vi "esp301 set position.vi"(7 "String":string, 8 "error in (no error)":errorcluster, 9 "Args":string[](array[string]), 10 "Seperator in":string, 11 "ESP301 in":refnum<class "ESP301.lvclass">) -> (0 "error out":errorcluster, 1 "s/mm":dbl=2.0, 2 "new commands":string, 3 "ESP301 out":refnum<class "ESP301.lvclass">, 5 "timeout":dbl)   [LabVIEW 2020, in "ESP301.lvclass"]
uses:
  ESP301.lvclass
  OnOffTypeDef.ctl
  ESP301.lvclass/ESP301.ctl
  openg_time.lvlib
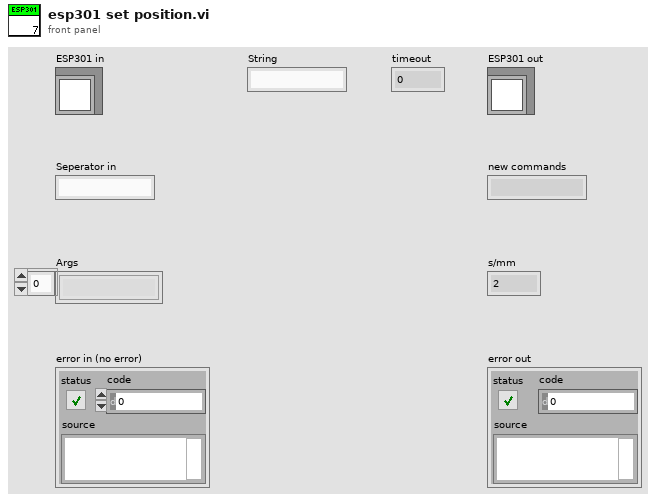
[diagram p1: front panel]
types:
  T1 = typedef "OnOffTypeDef.ctl" = enum16{"off", "on"}
  T2 = typedef "ESP301.lvclass/SettingsTypdef.ctl" = cluster{"devport":string, "Position":cluster{"Axis 1":cluster{"Value":dbl, "Min":dbl, "Max":dbl, "StepSize":dbl, "Tolerance":dbl, "ValueActual":dbl}, "Axis 2":cluster{"Value":dbl, "Min":dbl, "Max":dbl, "StepSize":dbl, "Tolerance":dbl, "ValueActual":dbl}, "Axis 3":cluster{"Value":dbl, "Min":dbl, "Max":dbl, "StepSize":dbl, "Tolerance":dbl, "ValueActual":dbl}}, "Power":cluster{"Axis 1":T1, "Axis 2":T1, "Axis 3":T1}, "Status":cluster{"Axis 1":T3, "Axis 2":T3, "Axis 3":T3}, "Backlash":cluster{"Axis 1":cluster{"Value":dbl, "Min":dbl, "Max":dbl, "StepSize":dbl, "Tolerance":dbl, "ValueActual":dbl}, "Axis 2":cluster{"Value":dbl, "Min":dbl, "Max":dbl, "StepSize":dbl, "Tolerance":dbl, "ValueActual":dbl}, "Axis 3":cluster{"Value":dbl, "Min":dbl, "Max":dbl, "StepSize":dbl, "Tolerance":dbl, "ValueActual":dbl}}, "Home":cluster{"Axis 1":cluster{"Value":dbl, "Min":dbl, "Max":dbl, "StepSize":dbl, "Tolerance":dbl, "ValueActual":dbl}, "Axis 2":cluster{"Value":dbl, "Min":dbl, "Max":dbl, "StepSize":dbl, "Tolerance":dbl, "ValueActual":dbl}, "Axis 3":cluster{"Value":dbl, "Min":dbl, "Max":dbl, "StepSize":dbl, "Tolerance":dbl, "ValueActual":dbl}}, "MoveToHardLimit":cluster{"Axis 1":T4, "Axis 2":T4, "Axis 3":T4}, "relativeMove":cluster{"Axis 1neg":T1, "Axis 2neg":T1, "Axis 3neg":T1, "Axis 1pos":T1, "Axis 2pos":T1, "Axis 3pos":T1}, "stepsize":cluster{"Value":dbl, "Min":dbl, "Max":dbl, "StepSize":dbl, "Tolerance":dbl, "ValueActual":dbl}, "automotoroff":T1, "ResetBeforeMove":T1, "Enable":cluster{"Axis 1":T1, "Axis 2":T1, "Axis 3":T1}}
  T3 = typedef "status_TypDef.ctl" = enum16{"Not referenced", "Homing", "Moving", "Ready"}
  T4 = typedef "Hardware limit.ctl" = enum16{"pos", "neg"}
  T5 = cluster{"Axis 1":cluster{"Value":dbl, "Min":dbl, "Max":dbl, "StepSize":dbl, "Tolerance":dbl, "ValueActual":dbl}, "Axis 2":cluster{"Value":dbl, "Min":dbl, "Max":dbl, "StepSize":dbl, "Tolerance":dbl, "ValueActual":dbl}, "Axis 3":cluster{"Value":dbl, "Min":dbl, "Max":dbl, "StepSize":dbl, "Tolerance":dbl, "ValueActual":dbl}}
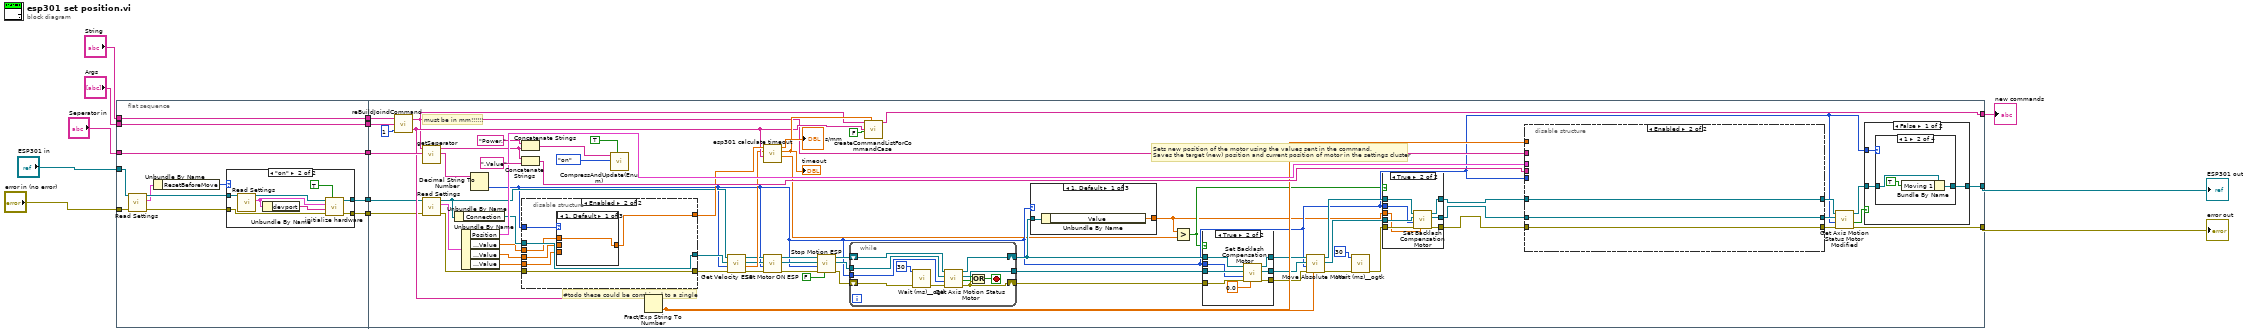
[diagram p0: block diagram]
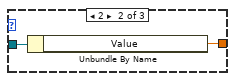
[diagram p3: hidden frame]
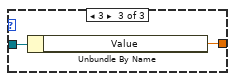
[diagram p4: hidden frame]
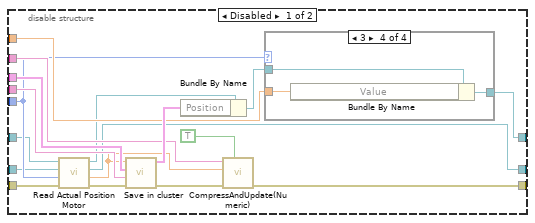
[diagram p7: hidden frame]
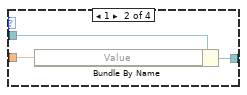
[diagram p9: hidden frame]
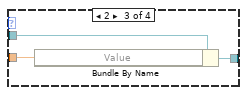
[diagram p10: hidden frame]
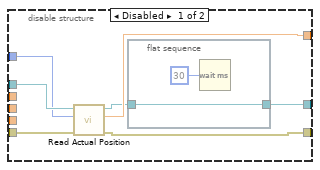
[diagram p11: hidden frame]
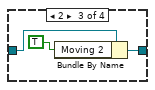
[diagram p15: hidden frame]
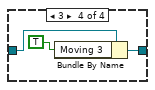
[diagram p16: hidden frame]
diagram:
  n1 = flat-sequence {
    tunnel: "error in (no error)" -> [w15]
    tunnel: "ESP301 in" -> [w14]
    tunnel: "Seperator in" -> [w22]
    tunnel: "String" -> [w23]
    tunnel: "Args" -> [w24]
    tunnel: [w24] -> w13
    tunnel: [w23] -> w12
    tunnel: [w22] -> w11
    tunnel: [w21] -> w10
    tunnel: [w20] -> w9
    tunnel: [w102] -> w1
    tunnel: [w61] -> w2
    tunnel: [w94] -> w6
    tunnel: w13 -> [w100]
    tunnel: w12 -> [w99]
    tunnel: w11 -> [w98]
    tunnel: w10 -> [w56]
    tunnel: w9 -> [w54]
    frame #0 {
      n2 = call-dynamic "Read Settings.vi"("error in (no error)"=w15, "ESP301 in"=w14) -> ("error out"=w16:errorcluster, "Settings"=w17:T2, "ESP301 out"=w18:refnum<class "ESP301.lvclass">)  [unwired: 7 in]
      n3 = Unbundle By Name(w17) -> ("ResetBeforeMove"=w19:T1)
      n4 = case shown="\"on\"" w19 {
        tunnel: [w26 w34] -> w21
        tunnel: w18 -> [w26 w29]
        tunnel: w16 -> [w25 w32]
        tunnel: [w25 w31] -> w20
        frame "off", Default {
        }
        frame "on" {
          n5 = call-dynamic "Read Settings.vi"("ESP301 in"=w29) -> ("Settings"=w27:T2, "ESP301 out"=w28:refnum<class "ESP301.lvclass">)  [unwired: 8 in, 1 out]
          n6 = Unbundle By Name(w27) -> ("devport"=w33:string)
          n7 = call-dynamic "initialize hardware.vi"("Reset (False)"=TRUE, "error in (no error)"=w32, "devport"=w33, "Settings"=w27, "ESP301 in"=w28) -> ("error out"=w31:errorcluster, "ESP301 out"=w34:refnum<class "ESP301.lvclass">)  [unwired: 4 in, 1 out]
        }
      }
    }
    frame #1 {
      # "#todo these could be combined to a single"
      # "must be in mm!!!!!!"
      # "Sets new position of the motor using the values sent in the command.\nSaves the target (new) position and current position of motor in the settings cluster"
      n8 = call "reBuildJoindCommand.vi"("number of group elements (0)"=1, "Args"=w100, "Command 2"=w99) -> ("Arg"=w82:string, "Command"=w81:string)
      n9 = call "getSeperator.vi"("Channel Seperator (\"\")"=w98, "Command"=w81) -> ("Channel"=w97:string, "Seperator (e.g. \"Channel1\")"=w89:string)  [unwired: 8 in]
      n10 = call-dynamic "Read Settings.vi"("error in (no error)"=w54, "ESP301 in"=w56) -> ("error out"=w55:errorcluster, "Settings"=w58:T2, "ESP301 out"=w57:refnum<class "ESP301.lvclass">)  [unwired: 7 in]
      n11 = Unbundle By Name(w57) -> ("Connection"=w85:refnum<visa-resource-name>)
      n12 = Unbundle By Name(w58) -> ("Position"=w92:T5, "Position.Axis 1.Value"=w53:dbl, "Position.Axis 2.Value"=w52:dbl, "Position.Axis 3.Value"=w51:dbl)
      n13 = Decimal String To Number(string=w97) -> (number=w41:i32)  [unwired: 2 in, 1 out]
      n14 = Concatenate Strings("Power." ("string"), w89) -> (w88:string)
      n15 = Concatenate Strings(w89, ".Value" ("string")) -> (w95:string)
      n16 = disable-structure shown="Enabled" {
        disable-tunnel: w85 -> [w168 w177]
        disable-tunnel: [w167 w175] -> w84
        disable-tunnel: [w162 w177] -> w79
        disable-tunnel: w55 -> [w166 w171]
        disable-tunnel: [w165 w171] -> w80
        disable-tunnel: w41 -> [w164 w176]
        disable-tunnel: w53 -> [_ w174]
        disable-tunnel: w52 -> [_ w173]
        disable-tunnel: w51 -> [_ w172]
        frame Disabled {
          n17 = call "Read Actual Position.vi"("error in (no error)"=w166, "Axis (1)"=w164, "VISA resource name"=w168) -> ("error out"=w165:errorcluster, "Position (units)"=w167:dbl, "VISA resource name out"=w163:refnum<visa-resource-name>)  [unwired: 2 in]
          n18 = flat-sequence {
            tunnel: w163 -> [w170]
            tunnel: [w170] -> w162
            frame #0 {
              n19 = Wait (ms)(milliseconds to wait=u32 30) -> ()  [unwired: 1 out]
            }
          }
        }
        frame Enabled {
          n20 = case shown="1, Default" w176 {
            tunnel: [w178 w179 w180] -> w175
            tunnel: w174 -> [w178 _ _]
            tunnel: w173 -> [_ w179 _]
            tunnel: w172 -> [_ _ w180]
            frame 1, Default {
            }
            frame 2 {
            }
            frame 3 {
            }
          }
        }
      }
      n21 = call "CompressAndUpdate(Enum).vi"("force CVT update (false)"=TRUE ("force CVT update"), "enum variant"=OnOffTypeDef."on" ("Axis 1"), "command or variable name"=w88) -> ()  [unwired: 8 in, 1 out]
      n22 = Fract/Exp String To Number(string=w82) -> (number=w67:dbl)  [unwired: 3 in, 1 out]
      n23 = call-dynamic "Get Velocity ESP.vi"("error in (no error)"=w80, "Axis (1)"=w41, "VISA resource name"=w79, "ESP301 in"=w57) -> ("error out"=w75:errorcluster, "Velocity (units/s)"=w78:dbl, "VISA resource name out"=w76:refnum<visa-resource-name>, "ESP301 out"=w77:refnum<class "ESP301.lvclass">)  [unwired: 4 in]
      n24 = call "esp301 calculate timeout.vi"("Arg"=w82, "Velocity (units/s)"=w78, "Position (units)"=w84) -> ("distance to move"=w40:dbl, "Numeric"=w83:dbl, "Numeric 2"=→"s/mm":dbl)  [unwired: 6 in]
      "timeout" <- w83
      n25 = call-dynamic "Set Motor ON ESP.vi"("error in (no error)"=w75, "Axis (1)"=w41, "VISA resource name"=w76, "ESP301 in"=w77) -> ("error out"=w74:errorcluster, "VISA resource name out"=w72:refnum<visa-resource-name>, "ESP301 out"=w69:refnum<class "ESP301.lvclass">)  [unwired: 5 in]
      n26 = call-dynamic "Stop Motion ESP.vi"("Stop all axes (F)"=FALSE, "error in (no error)"=w74, "Axis (1)"=w41, "VISA resource name"=w72, "ESP301 in"=w69) -> ("error out"=w70:errorcluster, "VISA resource name out"=w71:refnum<visa-resource-name>, "ESP301 out"=w68:refnum<class "ESP301.lvclass">)  [unwired: 4 in]
      n27 = while {
        tunnel: w71 -> [w204]
        tunnel: w41 -> [w200]
        tunnel: [w197] -> w49
        shift-right: [w202] -> w47
        shift-left: w70 -> [w203]
        shift-right: [w198] -> w42
        shift-left: w68 -> [w199]
        stop <- w205 stop-if-true
        n28 = call "Wait (ms)__ogtk.vi"("error in (no error)"=w203, "milliseconds to wait"=u32 30) -> ("error out"=w196:errorcluster)  [unwired: 8 in, 1 out]
        n29 = call-dynamic "Get Axis Motion Status Motor.vi"("error in (no error)"=w196, "Axis (1)"=w200, "VISA resource name"=w204, "ESP301 in"=w199) -> ("error out"=w202:errorcluster, "Motion Done"=w201:bool, "VISA resource name out"=w197:refnum<visa-resource-name>, "ESP301 out"=w198:refnum<class "ESP301.lvclass">)  [unwired: 4 in]
        n30 = Or(x=w201, y=w202) -> (x .or. y?=w205:bool)
      }
      n31 = call "createCommandListForCommandCase.vi"("timeout (optional)"=w83, "immediate Check (only once)"=FALSE, "setvalue"=w82, "command"=w81) -> ("new commands"=w102:string)  [unwired: 7 in]
      n32 = case shown="1, Default" w41 {
        tunnel: w42 -> [w104 w106 w108]
        tunnel: [w103 w105 w107] -> w38
        frame 1, Default {
          n33 = Unbundle By Name(w104) -> ("Value"=w103:dbl)
        }
        frame 2 {
          n34 = Unbundle By Name(w106) -> ("Value"=w105:dbl)
        }
        frame 3 {
          n35 = Unbundle By Name(w108) -> ("Value"=w107:dbl)
        }
      }
      n36 = Greater?(x=w38, y=w40) -> (0:w39:bool)
      n37 = case shown="True" w39 {
        tunnel: w42 -> [w122 w130]
        tunnel: [w122 w129] -> w50
        tunnel: w49 -> [w121 w128]
        tunnel: [w121 w127] -> w48
        tunnel: w41 -> [_ w126]
        tunnel: w47 -> [w120 w125]
        tunnel: [w120 w124] -> w46
        frame False {
        }
        frame True {
          n38 = call-dynamic "Set Backlash Compensation Motor.vi"("Backlash Compensation Value (0 units)"=0.0, "error in (no error)"=w125, "Axis (1)"=w126, "VISA resource name"=w128, "ESP301 in"=w130) -> ("error out"=w124:errorcluster, "VISA resource name out"=w127:refnum<visa-resource-name>, "ESP301 out"=w129:refnum<class "ESP301.lvclass">)  [unwired: 4 in]
        }
      }
      n39 = call-dynamic "Move Absolute Motor.vi"("Position (0 units)"=w67, "error in (no error)"=w46, "Axis (1)"=w41, "VISA resource name"=w48, "ESP301 in"=w50) -> ("error out"=w66:errorcluster, "VISA resource name out"=w45:refnum<visa-resource-name>, "ESP301 out"=w43:refnum<class "ESP301.lvclass">)  [unwired: 4 in]
      n40 = call "Wait (ms)__ogtk.vi"("error in (no error)"=w66, "milliseconds to wait"=u32 30) -> ("error out"=w44:errorcluster)  [unwired: 8 in, 1 out]
      n41 = case shown="True" w39 {
        tunnel: w43 -> [w111 w119]
        tunnel: [w111 w118] -> w37
        tunnel: w45 -> [w110 w117]
        tunnel: [w110 w116] -> w36
        tunnel: w41 -> [_ w115]
        tunnel: w44 -> [w109 w114]
        tunnel: [w109 w113] -> w35
        tunnel: w38 -> [_ w112]
        frame False {
        }
        frame True {
          n42 = call-dynamic "Set Backlash Compensation Motor.vi"("Backlash Compensation Value (0 units)"=w112, "error in (no error)"=w114, "Axis (1)"=w115, "VISA resource name"=w117, "ESP301 in"=w119) -> ("error out"=w113:errorcluster, "VISA resource name out"=w116:refnum<visa-resource-name>, "ESP301 out"=w118:refnum<class "ESP301.lvclass">)  [unwired: 4 in]
        }
      }
      n43 = disable-structure shown="Enabled" {
        disable-tunnel: [w148 w160] -> w62
        disable-tunnel: w95 -> [w147 _]
        disable-tunnel: [w131 w159] -> w60
        disable-tunnel: w36 -> [w134 w159]
        disable-tunnel: w35 -> [w138 w160]
        disable-tunnel: w92 -> [w145 _]
        disable-tunnel: [w142 w161] -> w64
        disable-tunnel: w67 -> [w141 _]
        disable-tunnel: w41 -> [w137 _]
        disable-tunnel: w81 -> [w139 _]
        disable-tunnel: w37 -> [w132 w161]
        frame Disabled {
          n44 = call-dynamic "Read Actual Position Motor.vi"("error in (no error)"=w138, "Axis (1)"=w137, "VISA resource name"=w134, "ESP301 in"=w132) -> ("error out"=w135:errorcluster, "Position (units)"=w136:dbl, "VISA resource name out"=w131:refnum<visa-resource-name>, "ESP301 out"=w133:refnum<class "ESP301.lvclass">)  [unwired: 4 in]
          n45 = call "Save in cluster.vi"("error in (no error)"=w135, "String"=w147, "Home in"=w145, "Numeric"=w136) -> ("error out"=w140:errorcluster, "Home out"=w144:T5)  [unwired: 6 in]
          n46 = Bundle By Name(cluster=w133, "Position"=w144) -> (w143:refnum<class "ESP301.lvclass">)
          n47 = call "CompressAndUpdate(Numeric).vi"("force CVT update (false)"=TRUE ("force CVT update"), "error in"=w140, "Numeric"=w136, "command or variable name"=w139) -> ("error out"=w148:errorcluster)  [unwired: 7 in]
          n48 = case shown="3" w137 {
            tunnel: w143 -> [w149 w152 w155 w158]
            tunnel: [w149 w151 w154 w157] -> w142
            tunnel: w141 -> [_ w150 w153 w156]
            frame 0, Default {
            }
            frame 1 {
              n49 = Bundle By Name(cluster=w152, "Value"=w150) -> (w151:refnum<class "ESP301.lvclass">)
            }
            frame 2 {
              n50 = Bundle By Name(cluster=w155, "Value"=w153) -> (w154:refnum<class "ESP301.lvclass">)
            }
            frame 3 {
              n51 = Bundle By Name(cluster=w158, "Value"=w156) -> (w157:refnum<class "ESP301.lvclass">)
            }
          }
        }
        frame Enabled {
        }
      }
      n52 = call-dynamic "Get Axis Motion Status Motor Modified.vi"("error in (no error)"=w62, "Axis (1)"=w41, "VISA resource name"=w60, "ESP301 in"=w64) -> ("error out"=w61:errorcluster, "Motion Done"=w59:bool, "ESP301 out"=w63:refnum<class "ESP301.lvclass">)  [unwired: 4 in, 1 out]
      n53 = case shown="False" w59 {
        tunnel: w41 -> [w183 _]
        tunnel: w63 -> [w182 w194]
        tunnel: [w181 w194] -> w94
        frame False {
          n54 = case shown="1" w183 {
            tunnel: w182 -> [w184 w187 w190 w193]
            tunnel: [w184 w186 w189 w192] -> w181
            frame 0, Default {
            }
            frame 1 {
              n55 = Bundle By Name(cluster=w187, "Moving 1"=TRUE) -> (w186:refnum<class "ESP301.lvclass">)
            }
            frame 2 {
              n56 = Bundle By Name(cluster=w190, "Moving 2"=TRUE) -> (w189:refnum<class "ESP301.lvclass">)
            }
            frame 3 {
              n57 = Bundle By Name(cluster=w193, "Moving 3"=TRUE) -> (w192:refnum<class "ESP301.lvclass">)
            }
          }
        }
        frame True {
        }
      }
    }
  }
  "ESP301 out" <- w6
  "error out" <- w2
  "new commands" <- w1
